vi "Kinesis - Simulated Hardware.vi"   [LabVIEW 2017]
uses:
  D:/upwork/Laser Measurement Tool/Laser/tests/KIM101/Thorlabs.MotionControl.DeviceManagerCLI.dll
  tests/KIM101/Thorlabs.MotionControl.DeviceManagerCLI.dll
panel:
  # "See Block Diagram For Instructions"
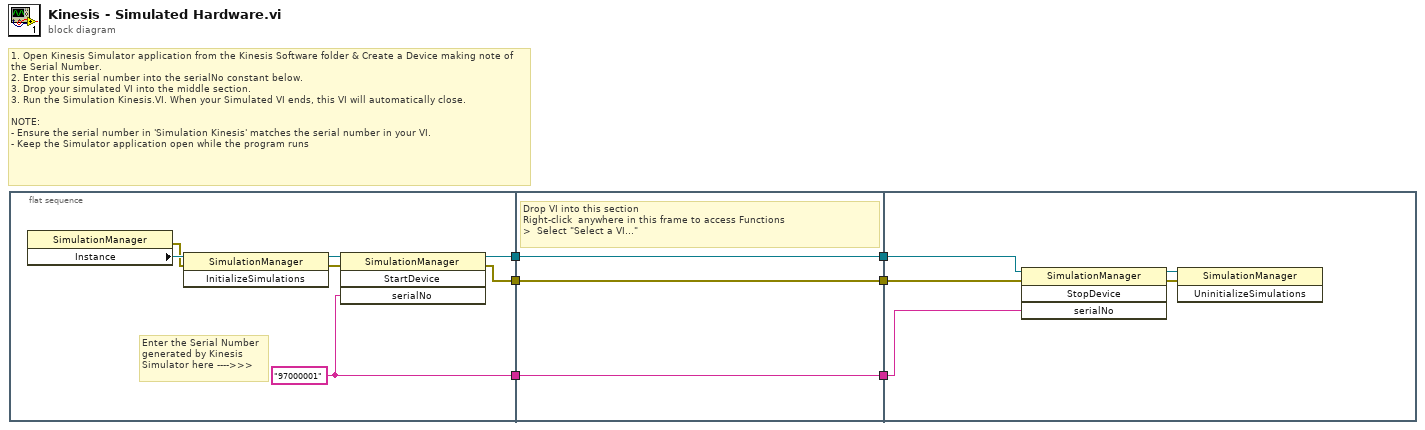
[diagram p0: block diagram]
diagram:
  # "1. Open Kinesis Simulator application from the Kinesis Software folder & Create a Device making note of the Serial Number.\n2. Enter this serial number into the serialNo constant below.\n3. Drop your simulated VI into the middle section.\n3. Run the Simulation Kinesis.VI. When your Simulated VI ends, this VI will automatically close.\n\nNOTE: \n- Ensure the serial number in 'Simulation Kinesis' matches the serial number in your VI.\n- Keep the Simulator application open while the program runs"
  n1 = flat-sequence {
    tunnel: [w11] -> w6
    tunnel: [w10] -> w3
    tunnel: [w7] -> w1
    tunnel: w6 -> [w16]
    tunnel: [w16] -> w5
    tunnel: [w15] -> w4
    tunnel: w3 -> [w15]
    tunnel: [w14] -> w2
    tunnel: w1 -> [w14]
    tunnel: w5 -> [w20]
    tunnel: w4 -> [w19]
    tunnel: w2 -> [w18]
    frame #0 {
      w11 = "97000001" ("serialNo")
      # "Enter the Serial Number\ngenerated by Kinesis \nSimulator here ---->>>"
      n2 = property class="SimulationManager"() -> (error out=w9:errorcluster, "Instance"=w13:refnum<k24>)  [unwired: 2 in, 1 out]
      n3 = invoke class="SimulationManager" method="InitializeSimulations"(reference=w13, error in=w9) -> (reference out=w12:refnum<k24>, error out=w8:errorcluster)  [unwired: 1 in, 1 out]
      n4 = invoke class="SimulationManager" method="StartDevice"(reference=w12, error in=w8, "serialNo"=w11) -> (reference out=w10:refnum<k24>, error out=w7:errorcluster)  [unwired: 1 in, 2 out]
    }
    frame #1 {
      # "Drop VI into this section\nRight-click  anywhere in this frame to access Functions \n>  Select \"Select a VI...\""
    }
    frame #2 {
      n5 = invoke class="SimulationManager" method="StopDevice"(reference=w19, error in=w18, "serialNo"=w20) -> (reference out=w21:refnum<k24>, error out=w17:errorcluster)  [unwired: 1 in, 2 out]
      n6 = invoke class="SimulationManager" method="UninitializeSimulations"(reference=w21, error in=w17) -> ()  [unwired: 1 in, 3 out]
    }
  }
